vi "Conditionally Throw Logger Not Initialized.vi"() -> (0 "error out":errorcluster)   [LabVIEW 2018, in "hse-logger.lvlib"]
doc: "A wrapper around the Error for the logger not being initialized. It covers three conditional disable symbols:\n- HSE_LOGGER_THROW_INIT_ERROR: throws error when no logger is initalized\n- HSE_LOGGER_THROW_INIT_WARNING: thorws a warning when no logger is initialized\n- default: does not throw any error"
uses:
  hse-logger.lvlib
panel:
  # "Connector Pane"
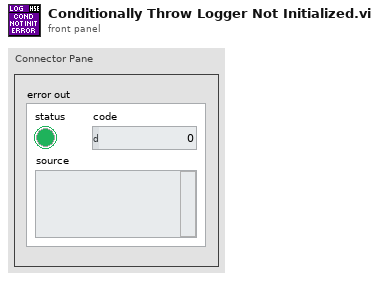
[diagram p1: front panel]
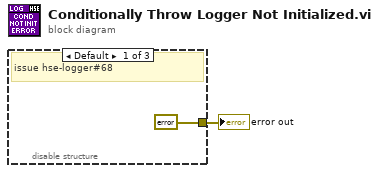
[diagram p0: block diagram]
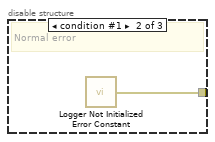
[diagram p2: hidden frame]
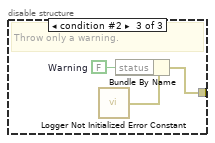
[diagram p3: hidden frame]
diagram:
  n1 = disable-structure shown="Default" {
    disable-tunnel: [errorcluster {"status"=FALSE, "code"=0, "source"=""} ("Logger Not Initialized Error") w3 w5] -> w1
    frame condition #0 (active) {
      # "issue hse-logger#68"
    }
    frame condition #1 {
      # "Normal error"
      n2 = call "Logger Not Initialized Error Constant.vi"() -> ("Logger Not Initialized Error"=w3:errorcluster)
    }
    frame condition #2 {
      w4 = FALSE  # Warning
      # "Throw only a warning."
      n3 = call "Logger Not Initialized Error Constant.vi"() -> ("Logger Not Initialized Error"=w6:errorcluster)
      n4 = Bundle By Name(cluster=w6, "status"=w4) -> (w5:errorcluster)
    }
  }
  "error out" <- w1
